vi "Get Status.vi"(8 "error in":T2, 11 "Communications Config":T1={"connection ID"=refnum, "IP"="192.168.0.108", "Active Comm Interface"=0, "Serial Port"="", "Programmer Type"=0, "connection ID"=refnum, "output cluster"={"GPIB address"=0, "GPIB bus"=0}} {"Programmer Type" items=["Model 430", "Model 420"]; "Active Comm Interface" items=["TCP/IP (Model 430 Only)", "RS232", "IEEE488"]}) -> (0 "error out":T2, 1 "state":T3=1 items=["Unknown", "RAMPING to target field/current", "HOLDING at the target field/current", "PAUSED", "Ramping in MANUAL UP mode", "Ramping in MANUAL DOWN mode", "ZEROING CURRENT (in progress)", "Quench detected", "At ZERO current", "Heating persistent switch", "Cooling persistent switch", "External Rampdown active"], 2 "Instrument Responded?":bool)   [LabVIEW 2017]
uses:
  Status AMI.ctl
  commsControl.ctl
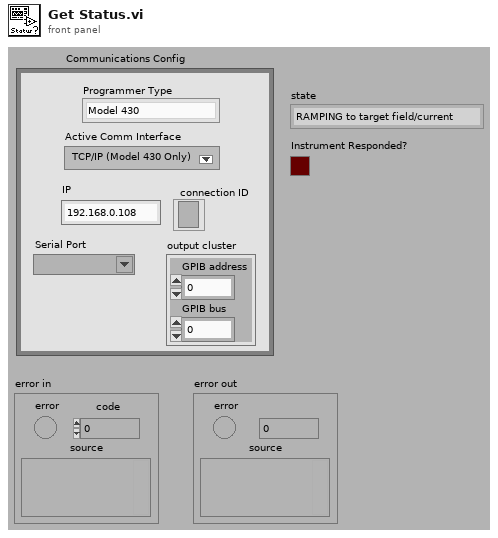
[diagram p1: front panel]
types:
  T1 = typedef "commsControl.ctl" = cluster{"connection ID":refnum<k5>, "IP":string, "Active Comm Interface":u16, "Serial Port":refnum<visa-resource-name>, "Programmer Type":u16, "connection ID":refnum<k5>, "output cluster":cluster{"GPIB address":i16, "GPIB bus":i16}}
  T2 = cluster{"error":bool, "code":i32, "source":string}
  T3 = typedef "Status AMI.ctl" = u16
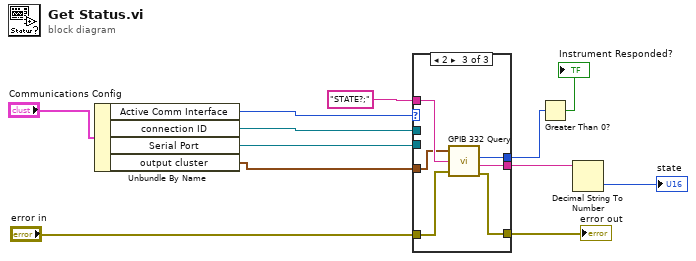
[diagram p0: block diagram]
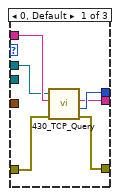
[diagram p2: hidden frame]
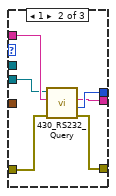
[diagram p3: hidden frame]
diagram:
  n1 = Unbundle By Name("Communications Config") -> ("Active Comm Interface"=w9:u16, "connection ID"=w8:refnum<k5>, "Serial Port"=w10:refnum<visa-resource-name>, "output cluster"=w1:cluster{"GPIB address":i16, "GPIB bus":i16})
  n2 = case shown="2" w9 {
    tunnel: "STATE?;" -> [w17 w23 w30]
    tunnel: "error in" -> [w13 w19 w29]
    tunnel: [w18 w24 w28] -> w5
    tunnel: [w15 w21 w26] -> w4
    tunnel: [w16 w22 w27] -> w3
    tunnel: w10 -> [_ w20 _]
    tunnel: w8 -> [w14 _ _]
    tunnel: w1 -> [_ _ w25]
    frame 0, Default {
      n3 = call "430_TCP_Query.vi"("error in (no error)"=w13, "Command"=w17, "connection ID"=w14) -> ("error out"=w18:errorcluster, "Bytes Read"=w16:i32, "Response"=w15:string)  [unwired: 4 in, 2 out]
    }
    frame 1 {
      n4 = call "430_RS232_Query.vi"("error in (no error)"=w19, "Command"=w23, "VISA resource name"=w20) -> ("error out"=w24:errorcluster, "Bytes Read"=w22:i32, "Response"=w21:string)  [unwired: 4 in, 2 out]
    }
    frame 2 {
      n5 = call "GPIB 332 Query.vi"("GPIB (In)"=w25, "Input query"=w30, "error in"=w29) -> ("Bytes returned"=w27:i32, "Return string"=w26:string, "error out"=w28:T2)  [unwired: 1 out]
    }
  }
  "error out" <- w5
  n6 = Greater Than 0?(x=w3) -> (x > 0?=→"Instrument Responded?":bool)
  n7 = Decimal String To Number(string=w4) -> (number=→"state":i32)  [unwired: 2 in, 1 out]
